vi "Demo.vi"() -> ()   [LabVIEW 2015]
uses:
  <vilib>/Stratom, Inc/X-CAN for myRIO (API)/X-CAN Class/Type Definitions/CANFrame.ctl
  Control/State.ctl
  <vilib>/Platform/TimedLoop/XDataNode/timing_clust.ctl
  <vilib>/Platform/TimedLoop/XDataNode/nitl_modes.ctl
  <vilib>/Platform/TimedLoop/XDataNode/wakeup.ctl
  <vilib>/Stratom, Inc/X-Modules for myRIO/Type Defs/MXPChannel.ctl
  <vilib>/Stratom, Inc/X-CAN for myRIO (API)/X-CAN Class/Type Definitions/CAN_Speed.ctl
  Control/Identifier.ctl
  <vilib>/Platform/TimedLoop/XDataNode/XDataNode.xnode
  <vilib>/Stratom, Inc/X-CAN for myRIO (API)/X-CAN Class/X-CAN.lvclass
  <vilib>/Platform/TimedLoop/XDataNode/XDNodeRunTimeDep.lvlib
panel:
  out "CAN Frame":T1 {"payload" format="%x"; "timestamp" format="%<%I:%M:%S%8u %p\n%x>T"; "identifier" format="%x"}
  in  "c_dec":bool
  in  "c_inc":bool
  out "Frequency(Hz)":dbl=0.5
  in  "Loop Rate [Hz]":u32(slide)=20 min=1 max=100 scale=1.0..100.0
  in  "Signal Type":enum16{"Sine", "Square", "Triangle"}(ring)
  in  "CAN Frame [Write]":cluster{"Identifier":u32, "Data Bytes":u8[]} {"Data Bytes" format="%x"; "Identifier" format="%x"}
  in  "Stop":bool
  in  "Write":bool
  out "Switch":bool[](array[boolean])
  out "Chart":u32(graph)
  in  "Freq_Index":u8=4
  # "NI myRIO X-CAN Demo"
  # "Data Transmit"
  # "Default Function"
  # "LCD Contrast"
  # "Data Received"
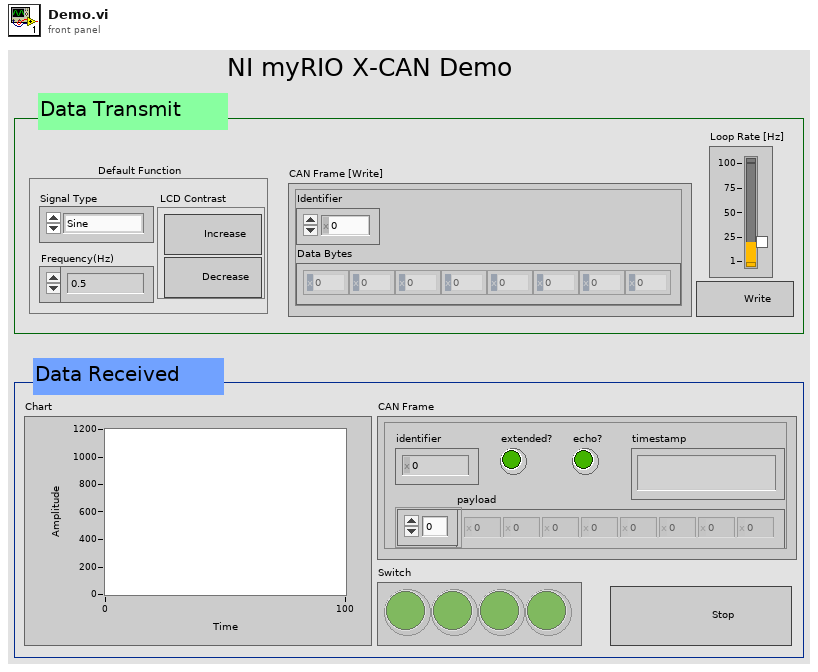
[diagram p1: front panel]
types:
  T1 = typedef "X-CAN.lvclass/CANFrame.ctl" = cluster{"identifier":u32, "extended?":bool, "echo?":bool, "payload":u8[], "timestamp":timestamp}
  T2 = typedef "State.ctl" = enum16{"Initialize", "Idle", "Write", "Stop"}
  T3 = typedef "XDNodeRunTimeDep.lvlib/timing_clust.ctl" = cluster{"Expected End [f-1]":u64, "Actual End [f-1]":u64, "Finished Late? [f-1]":bool, "Expected End [i-1]":u64, "Actual End [i-1]":u64, "Finished Late? [i-1]":bool, "Expected Start [i]":u64, "Actual Start [i]":u64, "Expected Start [f]":u64, "Actual Start [f]":u64, "Source Name":string, "Structure Name":string, "Period":i64, "Deadline":i64, "Offset":i64, "Start":i64, "Priority":i32, "Timeout":i32, "Mode":T4, "Wakeup Reason":T5, "Error":errorcluster, "Source Type":string, "Secondary Source Type":string, "Global End Time":u64, "Global Start Time":u64, "Frame Duration":u64, "Iteration Duration":u64, "Assigned CPU":i32, "I/O Scan Engine Mode":u32}
  T4 = typedef "XDNodeRunTimeDep.lvlib/nitl_modes.ctl" = enum32{"No Change", "Process missed periods, maintain original phase", "Discard missed periods, maintain original phase", "Process missed periods, ignore original phase", "Discard missed periods, ignore original phase"}
  T5 = typedef "XDNodeRunTimeDep.lvlib/wakeup.ctl" = enum32{"Normal", "Aborted", "Asynchronous wakeup", "Timing source error", "Timed loop error", "Timeout"}
  T6 = typedef "MXPChannel.ctl" = enum16{"A/MXP", "B/MXP"}
  T7 = typedef "Identifier.ctl" = enum16{"710"}
  T8 = typedef "X-CAN.lvclass/CAN_Speed.ctl" = u8
  T9 = cluster{"Signal Type":enum16{"Sine", "Square", "Triangle"}, "Freq_Index":u8, "c_inc":bool, "c_dec":bool, "Write":bool, "Stop":bool}
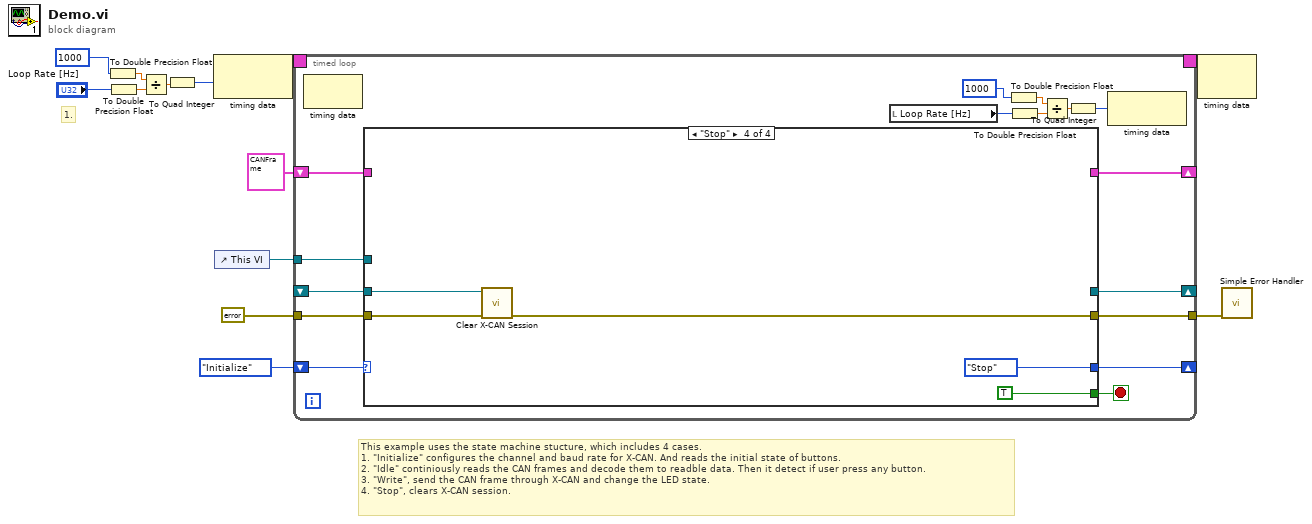
[diagram p0: block diagram]
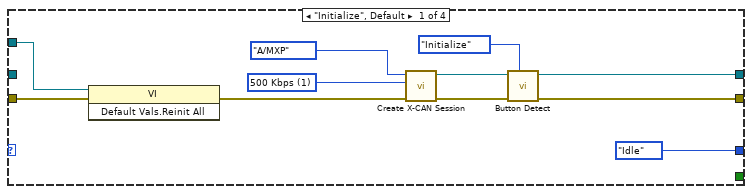
[diagram p2: hidden frame]
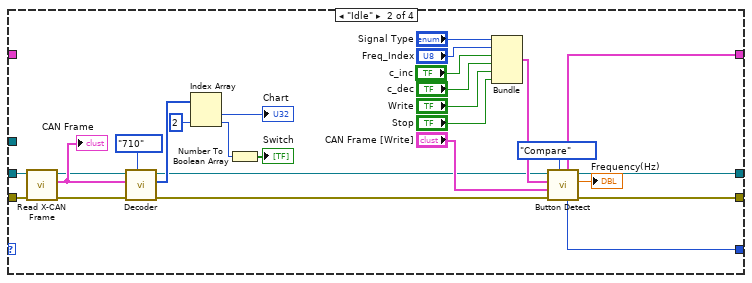
[diagram p3: hidden frame]
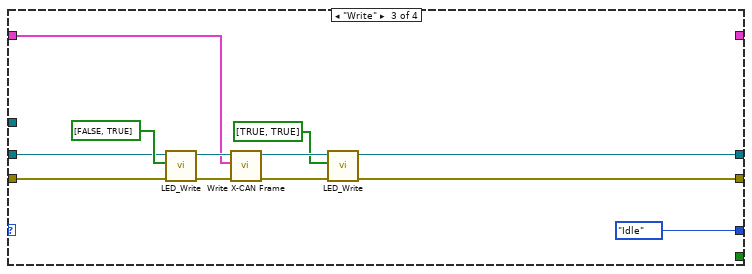
[diagram p4: hidden frame]
diagram:
  # "This example uses the state machine stucture, which includes 4 cases.\n1. \"Initialize\" configures the channel and baud rate for X-CAN. And reads the initial state of buttons.\n2. \"Idle\" continiously reads the CAN frames and decode them to readble data. Then it detect if user press any button.\n3. \"Write\", send the CAN frame through X-CAN and change the LED state.\n4. \"Stop\", clears X-CAN session."
  # "1."
  n1 = To Double Precision Float(number=u32 1000) -> (double precision float=w5:dbl)
  n2 = To Double Precision Float(number="Loop Rate [Hz]") -> (double precision float=w7:dbl)
  n3 = Divide(x=w5, y=w7) -> (x/y=w8:dbl)
  n4 = To Quad Integer(1:w8) -> (0:w3:i64)
  n5 = node-c288(w3) -> (w10:T3)
  n6 = control-ref of="This VI"() -> (w1:refnum<vi>)
  n7 = timed-loop {
    shift-right: [w28] -> _
    shift-left: State."Initialize" -> [w29]
    shift-right: [w15] -> _
    shift-left: T1 {"identifier"=0, "extended?"=FALSE, "echo?"=FALSE, "payload"=[0, 0, 0, 0, 0, 0, 0, 0], "timestamp"=timestamp(0 s since 1904-01-01)} ("CAN Frame [Write]") -> [w27]
    tunnel: [w26] -> w2
    tunnel: errorcluster {"status"=FALSE, "code"=0, "source"=""} ("error constant") -> [w25]
    shift-right: [w24] -> _
    shift-left: _ -> [w23]
    timing: w10 -> [_]
    timing-out: [_] -> w9
    tunnel: w1 -> [w14]
    stop <- w22 stop-if-true
    n8 = node-c288() -> ()  [unwired: 1 in, 1 out]
    n9 = case shown="\"Stop\"" w29 {
      tunnel: [State."Idle" w43 State."Idle" State."Stop"] -> w28
      tunnel: w27 -> [_ _ w72 _]
      tunnel: [w34 w67 w68 w82] -> w26
      tunnel: w25 -> [w42 w54 w70 w84]
      tunnel: [w35 w44 w69 _] -> w24
      tunnel: w23 -> [_ w55 w71 w83]
      tunnel: [_ _ _ TRUE] -> w22
      tunnel: [_ w66 _ _] -> w15
      tunnel: w14 -> [w36 _ _ _]
      frame "Initialize", Default {
        w40 = T8 1 items=["125 Kbps"=7, "250 Kbps"=3, "500 Kbps"=1, "1000 Kbps"=0, "95.238 Kbps"=6] ("CAN Speed [Kbps]")
        n10 = invoke class="VI" method="Default Vals.Reinit All"(reference=w36) -> ()  [unwired: 2 in, 3 out]
        n11 = call <vilib>:"Create X-CAN Session.vi"("error in (no error)"=w42, "CAN Speed [Kbps]"=w40, "MXP Channel"=MXPChannel."A/MXP") -> ("error out"=w38:errorcluster, "X-CAN Session out"=w35:refnum<class "X-CAN.lvclass">)  [unwired: 7 in]
        n12 = call "Button Detect.vi"("State"=enum16{"Initialize", "Compare"}."Initialize", "error in (no error)"=w38) -> ("error out"=w34:errorcluster)  [unwired: 6 in, 3 out]
      }
      frame "Idle" {
        n13 = call <vilib>:"Read X-CAN Frame.vi"("error in"=w54, "X-CAN Session in"=w55) -> ("error out"=w46:errorcluster, "CAN Frame"=w53:T1, "X-CAN Session out"=w44:refnum<class "X-CAN.lvclass">)  [unwired: 7 in]
        "CAN Frame" <- w53
        n14 = call "Decoder.vi"("Identifier"=Identifier."710", "error in (no error)"=w46, "CAN Frame"=w53) -> ("error out"=w45:errorcluster, "Output Data"=w51:u32[])  [unwired: 7 in]
        n15 = Index Array(array=w51, index #2=2 ("index")) -> (element #1=→"Chart":u32, element #2=w48:u32)  [unwired: 1 in]
        n16 = Number To Boolean Array(number=w48) -> (Boolean array=→"Switch":bool[])
        n17 = Bundle("Signal Type"="Signal Type", "Freq_Index"="Freq_Index", "c_inc"="c_inc", "c_dec"="c_dec", "Write"="Write", "Stop"="Stop") -> (w56:T9)  [unwired: 1 in]
        n18 = call "Button Detect.vi"("State"=enum16{"Initialize", "Compare"}."Compare", "error in (no error)"=w45, "CAN Frame [Write]"="CAN Frame [Write]", "output cluster"=w56) -> ("error out"=w67:errorcluster, "Freq"=→"Frequency(Hz)":dbl, "State Out"=w43:T2, "CAN Frame [Write] Out"=w66:T1)  [unwired: 4 in]
      }
      frame "Write" {
        n19 = call <vilib>:"LED_Write.vi"("error in"=w70, "LED Values"=bool[] [FALSE, TRUE], "X-CAN in"=w71) -> ("error out"=w77:errorcluster, "X-CAN out"=w74:refnum<class "X-CAN.lvclass">)  [unwired: 7 in]
        n20 = call <vilib>:"Write X-CAN Frame.vi"("error in"=w77, "CAN Frame"=w72, "X-CAN Session in"=w74) -> ("error out"=w76:errorcluster, "X-CAN Session out"=w75:refnum<class "X-CAN.lvclass">)  [unwired: 7 in]
        n21 = call <vilib>:"LED_Write.vi"("error in"=w76, "LED Values"=bool[] [TRUE, TRUE], "X-CAN in"=w75) -> ("error out"=w68:errorcluster, "X-CAN out"=w69:refnum<class "X-CAN.lvclass">)  [unwired: 7 in]
      }
      frame "Stop" {
        n22 = call <vilib>:"Clear X-CAN Session.vi"("error in (no error)"=w84, "X-CAN Session in"=w83) -> ("error out"=w82:errorcluster)  [unwired: 9 in]
      }
    }
    n23 = local read "Loop Rate [Hz]"() -> (w17:u32)
    n24 = To Double Precision Float(number=u32 1000) -> (double precision float=w21:dbl)
    n25 = To Double Precision Float(number=w17) -> (double precision float=w20:dbl)
    n26 = Divide(x=w21, y=w20) -> (x/y=w19:dbl)
    n27 = To Quad Integer(1:w19) -> (0:w16:i64)
    n28 = node-c288(w16) -> ()  [unwired: 1 out]
  }
  n29 = node-c288(w9) -> ()  [unwired: 1 out]
  n30 = call <vilib>:"Simple Error Handler.vi"("error in (no error)"=w2) -> ()  [unwired: 4 in, 5 out]
